vi "hse-application_DetermineConfigAndDataDirectories.vi"(8 "error in":errorcluster, 10 "Application Directory":path, 11 "Application Name":string) -> (0 "error out":errorcluster, 2 "Data Directory":path, 3 "Config Directory":path)   [LabVIEW 2020, in "hse-application.lvclass"]
doc: "Determines the paths of the _Config and _Data directories: \n- either by reading from the [HSE] section of <%APPNAME%>.ini in the application directory\n- or by defining them to live parallel to the application directory (this is HSE default)\n\n____\nHAMPEL SOFTWARE ENGINEERING v3.8.0 (2023-12-18 14:41)"
uses:
  hse-application.lvclass
  hse-configuration/config-ini/config-ini.lvclass
  hse-application.lvclass/hse-application.ctl
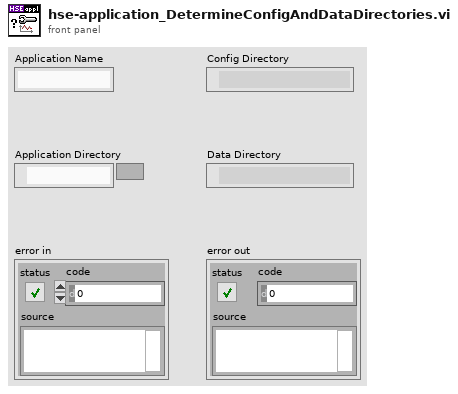
[diagram p1: front panel]
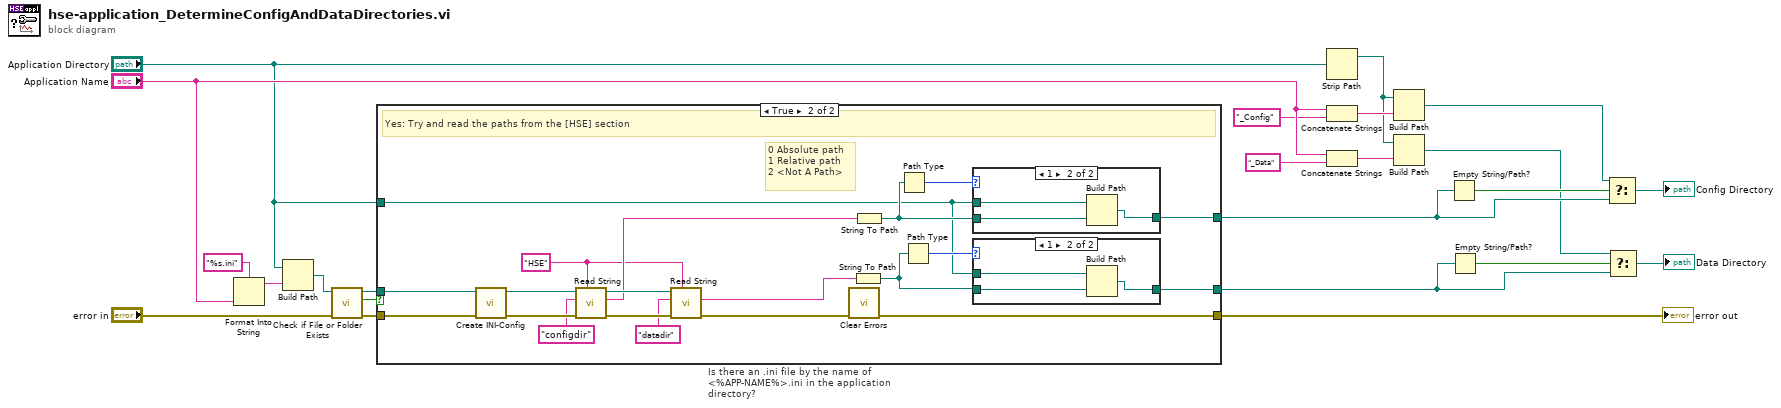
[diagram p0: block diagram]
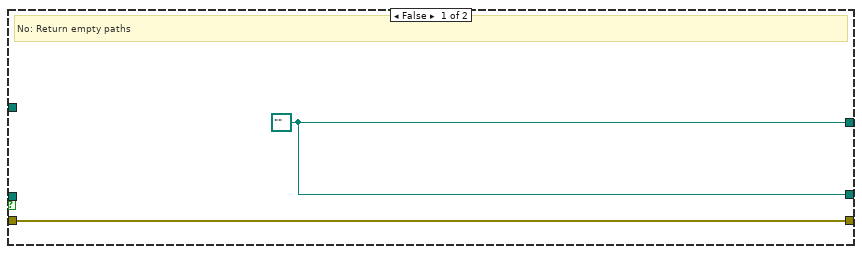
[diagram p2: hidden frame]
diagram:
  n1 = Format Into String(format string="%s.ini", "Application Name") -> (resulting string=w19:string)  [unwired: 2 in, 1 out]
  n2 = Build Path(base path="Application Directory", name or relative path=w19) -> (appended path=w18:path)
  n3 = call <vilib>:"Check if File or Folder Exists.vi"("error in (no error)"="error in", "path"=w18) -> ("error out"=w22:errorcluster, "file or folder exists?"=w17:bool, "dup path"=w16:path)  [unwired: 7 in]
  n4 = case "Is there an .ini file by the name of <%APP-NAME%>.ini in the application directory?" shown="True" w17 {
    tunnel: [w24 w32] -> w1
    tunnel: [w24 w34] -> w6
    tunnel: w16 -> [_ w29]
    tunnel: w22 -> [w25 w42]
    tunnel: [w25 w43] -> w21
    tunnel: "Application Directory" -> [_ w26]
    frame False {
      w24 = path "" ("appended path")
      # "No: Return empty paths"
    }
    frame True {
      w27 = "HSE" ("Section")
      # "0 Absolute path \n1 Relative path \n2 <Not A Path>"
      # "Yes: Try and read the paths from the [HSE] section"
      n5 = call "Create INI-Config.vi"("error in"=w42, "INI Filepath"=w29) -> ("error out"=w41:errorcluster, "config-ini out"=w28:refnum<class "config-ini.lvclass">)  [unwired: 8 in]
      n6 = call-dynamic "Read String.vi"("Section"=w27, "error in"=w41, "Key"="configdir", "config-base in"=w28) -> ("error out"=w45:errorcluster, "Value"=w36:string, "config-base out"=w38:refnum<class "config-ini.lvclass">)  [unwired: 5 in]
      n7 = call-dynamic "Read String.vi"("Section"=w27, "error in"=w45, "Key"="datadir", "config-base in"=w38) -> ("error out"=w44:errorcluster, "Value"=w37:string)  [unwired: 5 in, 1 out]
      n8 = call <vilib>:"Clear Errors.vi"("error in (no error)"=w44) -> ("error out"=w43:errorcluster)  [unwired: 5 in, 1 out]
      n9 = String To Path(string=w37) -> (path=w30:path)
      n10 = String To Path(string=w36) -> (path=w33:path)
      n11 = Path Type(1:w33) -> (0:w35:i16)
      n12 = Path Type(1:w30) -> (0:w31:i16)
      n13 = case shown="1" w35 {
        tunnel: [w50 w52] -> w34
        tunnel: w33 -> [w50 w53]
        tunnel: w26 -> [_ w51]
        frame 0, Default {
        }
        frame 1 {
          n14 = Build Path(base path=w51, name or relative path=w53) -> (appended path=w52:path)
        }
      }
      n15 = case shown="1" w31 {
        tunnel: [w46 w48] -> w32
        tunnel: w30 -> [w46 w49]
        tunnel: w26 -> [_ w47]
        frame 0, Default {
        }
        frame 1 {
          n16 = Build Path(base path=w47, name or relative path=w49) -> (appended path=w48:path)
        }
      }
    }
  }
  "error out" <- w21
  n17 = Strip Path(path="Application Directory") -> (stripped path=w10:path)  [unwired: 1 out]
  n18 = Concatenate Strings("Application Name", "_Config" ("Substring")) -> (w11:string)
  n19 = Concatenate Strings("Application Name", "_Data" ("Substring")) -> (w9:string)
  n20 = Build Path(base path=w10, name or relative path=w11) -> (appended path=w7:path)
  n21 = Build Path(base path=w10, name or relative path=w9) -> (appended path=w3:path)
  n22 = Empty String/Path?(string/path=w6) -> (empty?=w8:bool)
  n23 = Empty String/Path?(string/path=w1) -> (empty?=w4:bool)
  n24 = Select(t=w7, s=w8, f=w6) -> (s? t:f=→"Config Directory":path)
  n25 = Select(t=w3, s=w4, f=w1) -> (s? t:f=→"Data Directory":path)
